vi "linear fit of widths.vi"() -> ()   [LabVIEW 2016]
uses:
  <vilib>/Analysis/baseanly.llb/Mean (DBL).vi
  <vilib>/Analysis/6fits.llb/Remove Outliers (Range).vi
  <vilib>/Analysis/NI_AALBase.lvlib
  <vilib>/Analysis/NI_AALPro.lvlib
panel:
  out "0.037 fake data with noise 3":cluster{"X Out":dbl[], "Y Out":dbl[]}(graph)
  out "intercept":dbl=0.003467464780820419
  out "slope":dbl=-0.006836565246472789
  in  "Range":dbl[](array[numeric])
  out "mean":dbl=0.04032457952734193 format="%e"
  out "0.037 fake data with noise 2":T1(graph)
  in  "length":i32=43
  in  "index":i32=60
  in  "width":cluster{dbl[], dbl[]}[](graph)
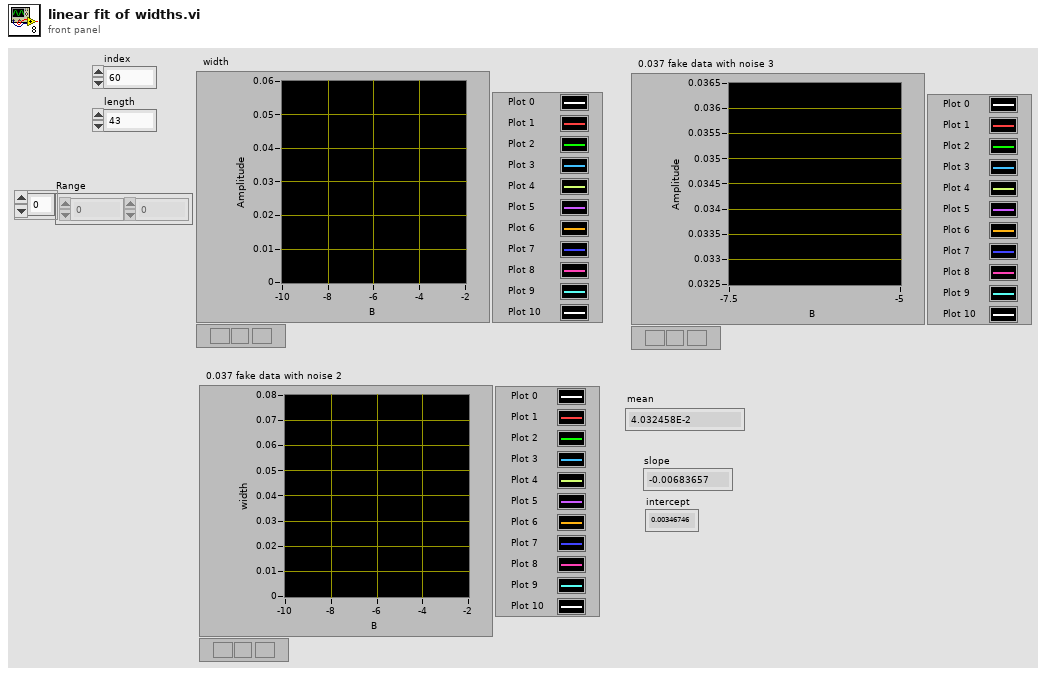
[diagram p1: front panel]
types:
  T1 = cluster{"X Out":dbl[], "Best Linear Fit":dbl[]}[]
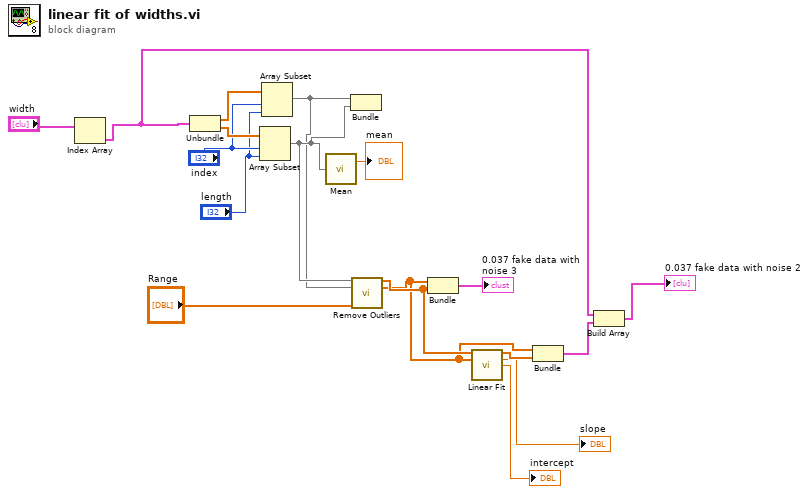
[diagram p0: block diagram]
diagram:
  n1 = Index Array(array="width") -> (element=w1:cluster{dbl[], dbl[]})  [unwired: 1 in]
  n2 = Unbundle(w1) -> (w17:dbl[], w18:dbl[])
  n3 = Array Subset(array=w18, index="index", length="length") -> (w12:dbl[])
  n4 = Array Subset(array=w17, index="index", length="length") -> (w11:dbl[])
  n5 = call-poly <vilib>:"Mean.vi"("X"=w12) -> ("mean"=→"mean":dbl)  [unwired: 1 out]
  n6 = Bundle(w11, w12) -> ()  [unwired: 1 in, 1 out]
  n7 = call-poly <vilib>:"Remove Outliers.vi"("Y"=w12, "X"=w11, "Range"="Range") -> ("Y Out"=w10:dbl[], "X Out"=w8:dbl[])  [unwired: 8 in, 3 out]
  n8 = Bundle("X Out"=w8, "Y Out"=w10) -> (→"0.037 fake data with noise 3":cluster{"X Out":dbl[], "Y Out":dbl[]})  [unwired: 1 in]
  n9 = call <vilib>:"Linear Fit.vi"("Y"=w10, "X"=w8) -> ("Best Linear Fit"=w9:dbl[], "slope"=→"slope":dbl, "intercept"=→"intercept":dbl)  [unwired: 9 in, 2 out]
  n10 = Bundle("X Out"=w8, "Best Linear Fit"=w9) -> (w7:cluster{"X Out":dbl[], "Best Linear Fit":dbl[]})  [unwired: 1 in]
  n11 = Build Array(w1, w7) -> (→"0.037 fake data with noise 2":T1)
